vi "HWT_Shared_Proc_Initialize.vi"(8 "error in (no error)":errorcluster, 11 "Q-Name":string) -> (0 "error out":errorcluster, 3 "Queue out":refnum<queue>)   [LabVIEW 2015]
uses:
  Controls/Control_General Command Cluster.ctl
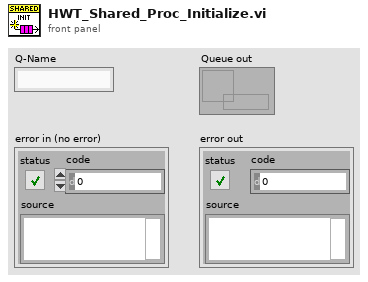
[diagram p1: front panel]
types:
  T1 = typedef "Control_General Command Cluster.ctl" = cluster{"Caller-Q":refnum<queue>, "Command":string, "Return":string, "Data":variant, "Timeout":dbl}
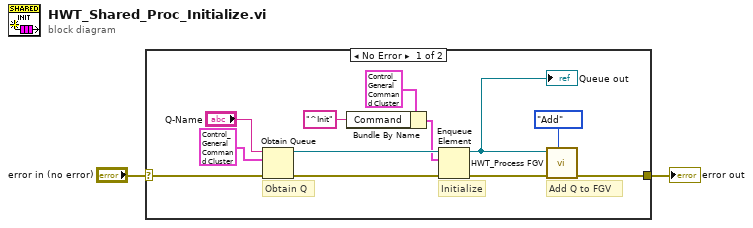
[diagram p0: block diagram]
diagram:
  n1 = case shown="No Error" "error in (no error)" {
    selector: "error in (no error)" -> [w7 w15]
    tunnel: [w5 w15] -> w1
    frame No Error {
      # "Add Q to FGV"
      # "Initialize"
      # "Obtain Q"
      n2 = Obtain Queue(name (unnamed)="Q-Name", element data type=T1 {"Caller-Q"=refnum, "Command"="", "Return"="", "Data"=variant, "Timeout"=0.0}, error in (no error)=w7) -> (queue out=w13:refnum<queue>, error out=w8:errorcluster)  [unwired: 2 in, 1 out]
      n3 = Bundle By Name(cluster=T1 {"Caller-Q"=refnum, "Command"="", "Return"="", "Data"=variant, "Timeout"=0.0}, "Command"="^Init") -> (w12:T1)
      n4 = Enqueue Element(queue=w13, element=w12, error in (no error)=w8) -> (queue out=w4:refnum<queue>, error out=w6:errorcluster)  [unwired: 1 in, 1 out]
      "Queue out" <- w4
      n5 = call "HWT_Process FGV.vi"("Action"=enum16{"Init", "Add", "Get"}."Add", "error in (no error)"=w6, "Queue in"=w4) -> ("error out"=w5:errorcluster)  [unwired: 7 in, 1 out]
    }
    frame Error {
    }
  }
  "error out" <- w1
